vi "CRYMouse Down in Graph Window.vi"(6 "Queue":refnum<queue>, 8 "Event Name":string, 9 "Selected Type":enum16{"Curves", "Values", "Results", "WFM"}(ring), 11 "pGraph VI In":refnum<vi>) -> (0 "Type Out":enum16{"Curves", "Values", "Results", "WFM"}(ring))   [LabVIEW 2013]
uses:
  CRYCurveLibrary/Global/CRYCurve Library Global.vi
panel:
  out "Queue Name":string
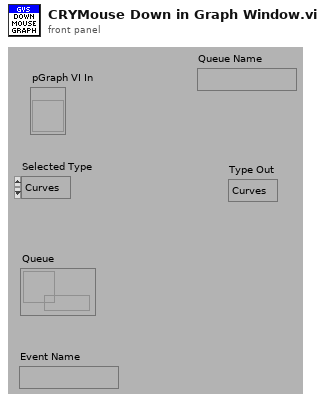
[diagram p1: front panel]
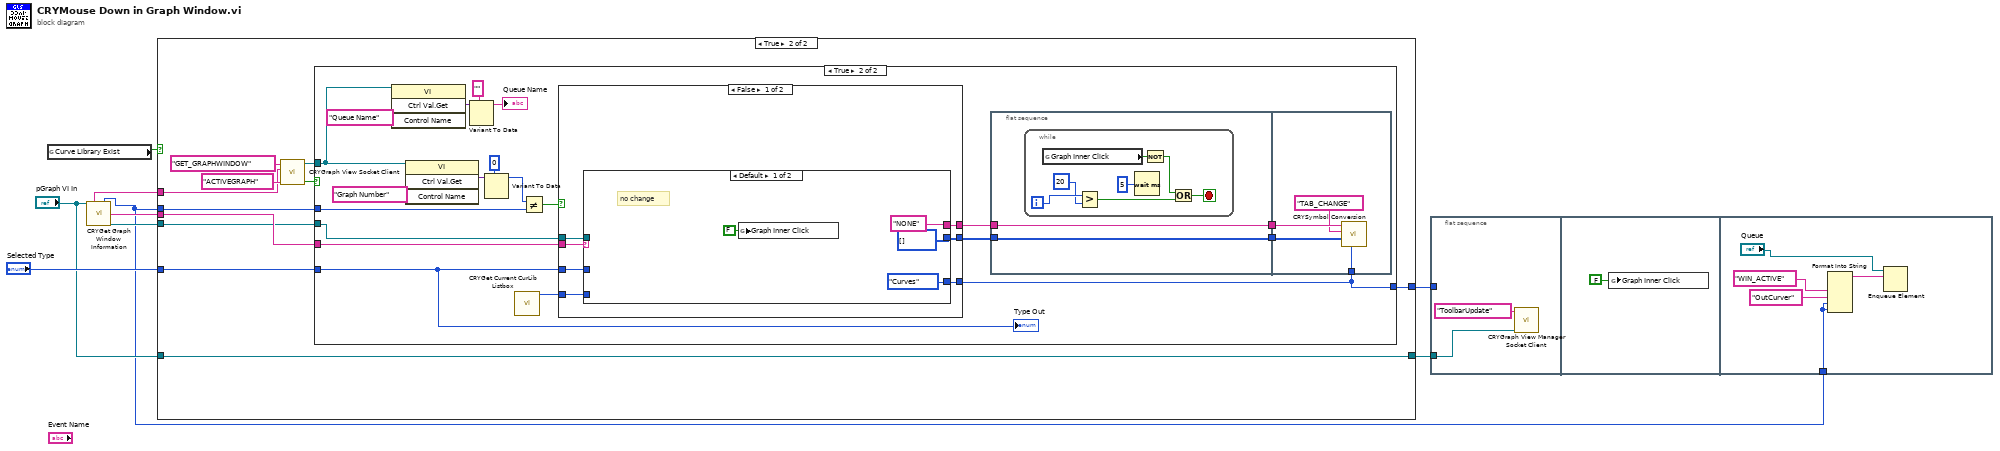
[diagram p0: block diagram]
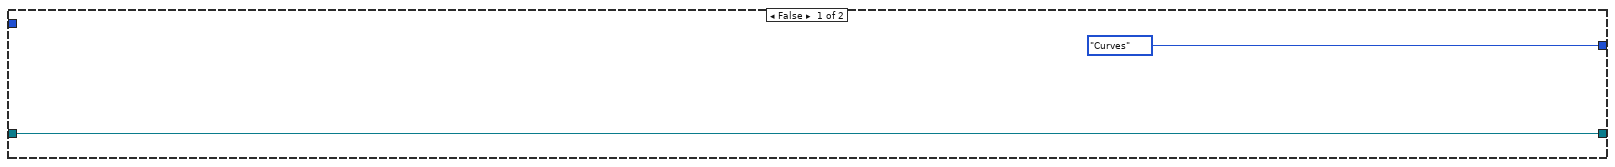
[diagram p2: hidden frame]
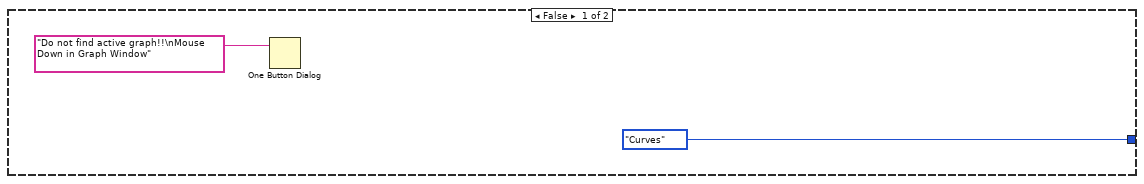
[diagram p3: hidden frame]
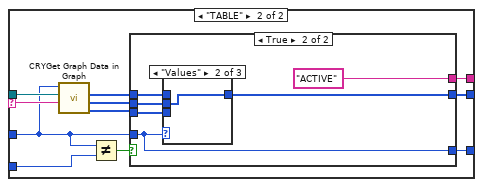
[diagram p4: hidden frame]
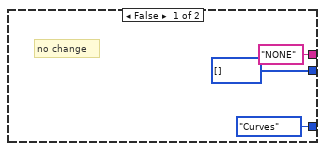
[diagram p5: hidden frame]
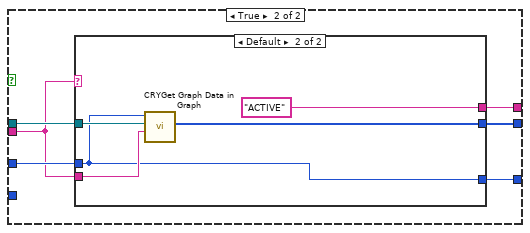
[diagram p8: hidden frame]
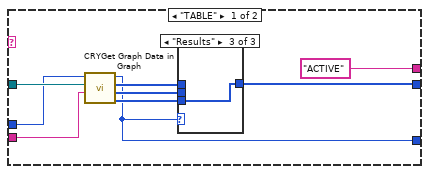
[diagram p9: hidden frame]
diagram:
  n1 = global read "CRYCurve Library Global.vi" "Curve Library Exist"() -> (w5:bool)
  n2 = call "CRYGet Graph Window Information.vi"("pGraph VI In"="pGraph VI In") -> ("Queue Name Out"=w6:string, "Graph Number Out"=w1:i32, "Graph Type Out"=w7:string, "Legend Ref Out"=w8:refnum<vi>)  [unwired: 4 in, 7 out]
  n3 = case shown="True" w5 {
    tunnel: "Selected Type" -> [_ w22]
    tunnel: w8 -> [_ w13]
    tunnel: w7 -> [_ w21]
    tunnel: w1 -> [_ w17]
    tunnel: w6 -> [_ w16]
    tunnel: [enum16{"Curves", "Values", "Results", "WFM"}."Curves" ("Selected Type") w15] -> w4
    tunnel: [w10 w12] -> w3
    tunnel: "pGraph VI In" -> [w10 w12]
    frame False {
    }
    frame True {
      n4 = call "CRYGraph View Socket Client.vi"("sOption"="ACTIVEGRAPH", "sData"=w16, "sAction"="GET_GRAPHWINDOW") -> ("bResult Out"=w14:bool, "pVI Out"=w18:refnum<vi>)  [unwired: 5 in, 2 out]
      n5 = case shown="True" w14 {
        tunnel: w22 -> [_ w44]
        tunnel: w13 -> [_ w43]
        tunnel: w21 -> [_ w42]
        tunnel: w18 -> [_ w31]
        tunnel: w17 -> [_ w39]
        tunnel: [enum16{"Curves", "Values", "Results", "WFM"}."Curves" ("Selected Type") w36] -> w15
        frame False {
          n6 = One Button Dialog(message="Do not find active graph!!\nMouse Down in Graph Window") -> ()  [unwired: 1 in, 1 out]
        }
        frame True {
          n7 = invoke class="VI" method="Ctrl Val.Get"(reference=w31, "Control Name"="Queue Name" ("input 1")) -> ("Get Control Value Variant"=w29:variant)  [unwired: 2 in, 3 out]
          n8 = invoke class="VI" method="Ctrl Val.Get"(reference=w31, "Control Name"="Graph Number") -> ("Get Control Value Variant"=w34:variant)  [unwired: 2 in, 3 out]
          n9 = Variant To Data(type="" ("input 1"), Variant=w29) -> (data=→"Queue Name":string)  [unwired: 1 in, 1 out]
          n10 = Variant To Data(type=0 ("Graph Number"), Variant=w34) -> (data=w32:i32)  [unwired: 1 in, 1 out]
          n11 = call "CRYGet Current CurLib Listbox.vi"() -> ("Type"=w41:enum16{"Curves", "Values", "Results", "WFM"})  [unwired: 9 in, 2 out]
          n12 = Not Equal?(x=w32, y=w39) -> (x != y?=w40:bool)
          n13 = case shown="False" w40 {
            tunnel: w43 -> [w63 w97]
            tunnel: w44 -> [w62 w96]
            tunnel: w42 -> [w64 w95]
            tunnel: w41 -> [w61 _]
            tunnel: [w60 w94] -> w38
            tunnel: [w59 w93] -> w37
            tunnel: [w58 w92] -> w36
            frame False {
              n14 = case shown="Default" w64 {
                selector: w64 -> [_ w78]
                tunnel: w63 -> [_ w79]
                tunnel: w62 -> [_ w75]
                tunnel: w61 -> [_ w76]
                tunnel: [i32[] [] ("Result Rows") w71] -> w60
                tunnel: ["NONE" ("sActin") w70] -> w59
                tunnel: [enum16{"Curves", "Values", "Results", "WFM"}."Curves" ("Selected Type") w69] -> w58
                frame Default {
                  # "no change"
                  n15 = global write "CRYCurve Library Global.vi" "Graph Inner Click"(FALSE ("Graph Inner Click")) -> ()
                }
                frame "TABLE" {
                  n16 = call "CRYGet Graph Data in Graph.vi"("Graph Type"=w78, "Legend Refnum"=w79, "Type In"=w75) -> ("Result Rows"=w72:i32[], "Value Rows"=w73:i32[], "Rows"=w77:i32[])  [unwired: 1 in, 5 out]
                  n17 = Not Equal?(x=w75, y=w76) -> (x != y?=w74:bool)
                  n18 = case shown="True" w74 {
                    tunnel: w77 -> [_ w88]
                    tunnel: w75 -> [_ w83]
                    tunnel: w73 -> [_ w87]
                    tunnel: w72 -> [_ w86]
                    tunnel: [i32[] [] ("Result Rows") w85] -> w71
                    tunnel: ["NONE" ("sActin") "ACTIVE" ("sActin")] -> w70
                    tunnel: [enum16{"Curves", "Values", "Results", "WFM"}."Curves" ("Selected Type") w83] -> w69
                    frame False {
                      # "no change"
                    }
                    frame True {
                      n19 = case shown="\"Values\"" w83 {
                        tunnel: w88 -> [w89 _ _]
                        tunnel: w87 -> [_ w90 _]
                        tunnel: w86 -> [_ _ w91]
                        tunnel: [w89 w90 w91] -> w85
                        frame "Curves", Default {
                        }
                        frame "Values" {
                        }
                        frame "Results" {
                        }
                      }
                    }
                  }
                }
              }
            }
            frame True {
              n20 = case shown="Default" w95 {
                tunnel: w97 -> [w106 w114]
                tunnel: w96 -> [w103 w111]
                tunnel: w95 -> [w105 w113]
                tunnel: [w100 w110] -> w94
                tunnel: ["ACTIVE" ("sActin") "ACTIVE" ("sActin")] -> w93
                tunnel: [w98 w111] -> w92
                frame "TABLE" {
                  n21 = call "CRYGet Graph Data in Graph.vi"("Graph Type"=w105, "Legend Refnum"=w106, "Type In"=w103) -> ("Result Rows"=w101:i32[], "Value Rows"=w102:i32[], "Rows"=w104:i32[], "Type Out"=w98:enum16{"Curves", "Values", "Results", "WFM"})  [unwired: 1 in, 4 out]
                  n22 = case shown="\"Results\"" w98 {
                    tunnel: w104 -> [w107 _ _]
                    tunnel: w102 -> [_ w108 _]
                    tunnel: w101 -> [_ _ w109]
                    tunnel: [w107 w108 w109] -> w100
                    frame "Curves", Default {
                    }
                    frame "Values" {
                    }
                    frame "Results" {
                    }
                  }
                }
                frame Default {
                  n23 = call "CRYGet Graph Data in Graph.vi"("Graph Type"=w113, "Legend Refnum"=w114, "Type In"=w111) -> ("Rows"=w110:i32[])  [unwired: 1 in, 7 out]
                }
              }
            }
          }
          n24 = flat-sequence {
            tunnel: w37 -> [w45]
            tunnel: w38 -> [w46]
            tunnel: [w46] -> w26
            tunnel: [w45] -> w25
            tunnel: w36 -> [w55]
            tunnel: w26 -> [w57]
            tunnel: w25 -> [w56]
            frame #0 {
              n25 = while {
                i -> [w48]
                stop <- w50 stop-if-true
                n26 = global read "CRYCurve Library Global.vi" "Graph Inner Click"() -> (w53:bool)
                n27 = Greater?(x=w48, y=20) -> (0:w51:bool)
                n28 = Wait (ms)(milliseconds to wait=u32 5) -> ()  [unwired: 1 out]
                n29 = Not(x=w53) -> (.not. x?=w52:bool)
                n30 = Or(x=w52, y=w51) -> (x .or. y?=w50:bool)
              }
            }
            frame #1 {
              n31 = call "CRYSymbol Conversion.vi"("CurLib Tab Type"=w55, "nDatas"=w57, "sData"="TAB_CHANGE" ("sActin"), "sActin"=w56) -> ()  [unwired: 8 in]
            }
          }
          "Type Out" <- w44
        }
      }
    }
  }
  n32 = flat-sequence {
    tunnel: w4 -> [_]
    tunnel: w3 -> [w116]
    tunnel: w1 -> [w118]
    frame #0 {
      n33 = call "CRYGraph View Manager Socket Client.vi"("pVI Ref"=w116, "sAction"="ToolbarUpdate") -> ()  [unwired: 10 in]
    }
    frame #1 {
      n34 = global write "CRYCurve Library Global.vi" "Graph Inner Click"(FALSE ("Graph Inner Click")) -> ()
    }
    frame #2 {
      n35 = Format Into String("WIN_ACTIVE" ("input 1"), "OutCurver" ("input 1"), w118, w118) -> (resulting string=w120:string)  [unwired: 3 in, 1 out]
      n36 = Enqueue Element(queue="Queue", element=w120) -> ()  [unwired: 1 in, 4 out]
    }
  }
